vi "Collect_Coordinates(X,Y)_in_Array.vi"(2 "Initial Index \nfor Replacement":i32, 3 "[IN] Array for \nCollecting \nCoord (X,Y)":dbl[](array[numeric]), 4 "Y":dbl, 5 "X":dbl) -> (0 "Finish\nIndex":i32, 1 "[OUT] Array\nfor collecting":dbl[](array[numeric]))   [LabVIEW 2013]
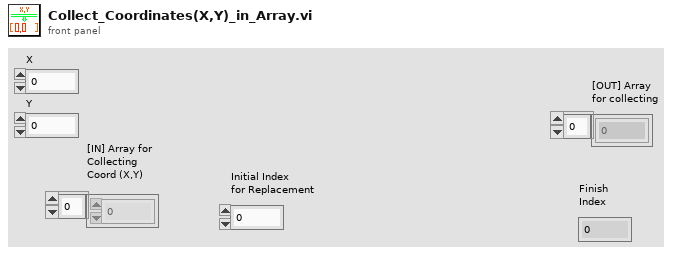
[diagram p1: front panel]
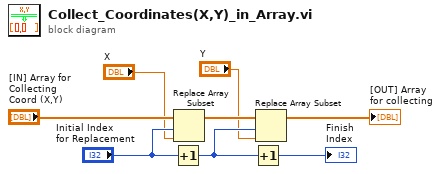
[diagram p0: block diagram]
diagram:
  n1 = Increment(x="Initial Index \nfor Replacement") -> (x+1=w7:i32)
  n2 = Replace Array Subset(array="[IN] Array for \nCollecting \nCoord (X,Y)", new element="X", index="Initial Index \nfor Replacement") -> (w8:dbl[])
  n3 = Increment(x=w7) -> (x+1=→"Finish\nIndex":i32)
  n4 = Replace Array Subset(array=w8, new element="Y", index=w7) -> (→"[OUT] Array\nfor collecting":dbl[])
